vi "Read Dashboard Variables.vi"() -> ()   [LabVIEW 2019]
uses:
  <vilib>/Rock Robotics/Network Tables/NT Read Number.vi
  Framework/Robot Global Data.vi
  <vilib>/Rock Robotics/Network Tables/NT Read String.vi
  <vilib>/Rock Robotics/Network Tables/NT Read Boolean.vi
panel:
  out "Speed Rate at 2 inches":dbl
  out "Speed Rate at 6 inches":dbl
  out "Data Logger":bool
  out "Pivot Right R":dbl=0.4
  out "Pivot Right L":dbl=0.3
  out "Pivot Left R":dbl=0.4
  out "Pivot Left L":dbl=0.3
  out "Path":string
  out "MaxSpeedSlow":dbl=0.6
  out "Intake Set Point":dbl=1.0
  out "Intake Duration":dbl=0.5
  out "Shooter Set Point":dbl=1.0
  out "Shooter Duration":dbl=0.5
  out "Transfer Set Point":dbl=0.6
  out "Transfer Duration":dbl=0.5
  out "Control Panel Set Point":dbl=0.6
  out "Control Panel Duration":dbl=5.5
  out "Control Panel Color Set Point":dbl=0.3
  out "Control Panel Color Duration":dbl=4.0
  out "MaxDrive":dbl(slide)=1.0 min=0.0 max=1.0 step=0.01 scale=0.0..1.0
  out "DriveK":dbl(slide)=0.5 min=0.0 max=1.0 step=0.05 scale=0.0..1.0
  out "Limelight Goal Area":dbl(slide)=1.91 min=0.1 max=2.5 step=0.25 scale=0.0..2.5
  out "MinSteerCommand":dbl(slide)=0.2717391304347826 min=0.0 max=0.5 step=0.05 scale=0.0..0.5
  out "SteeringK":dbl(slide)=0.025362318840579712 min=0.0 max=0.25 step=0.01 scale=0.0..0.25
  out "AimDeadband":dbl=0.1 min=0.0 max=10.0 step=0.25
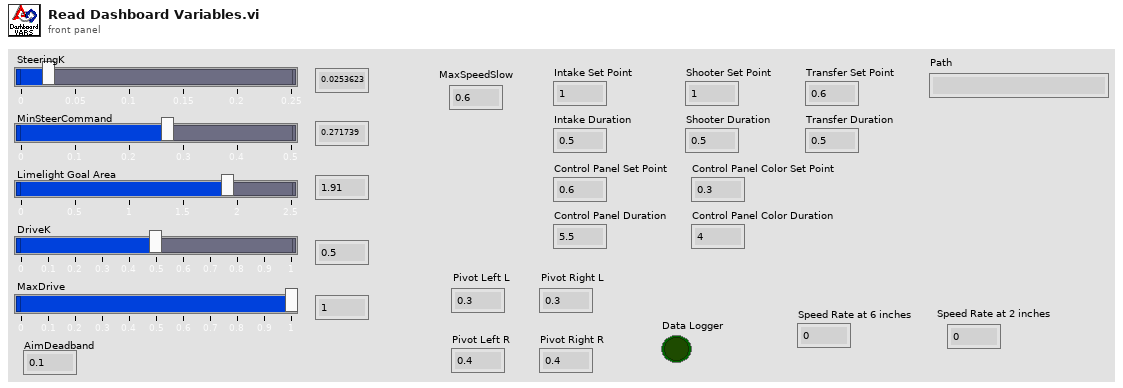
[diagram p1: front panel]
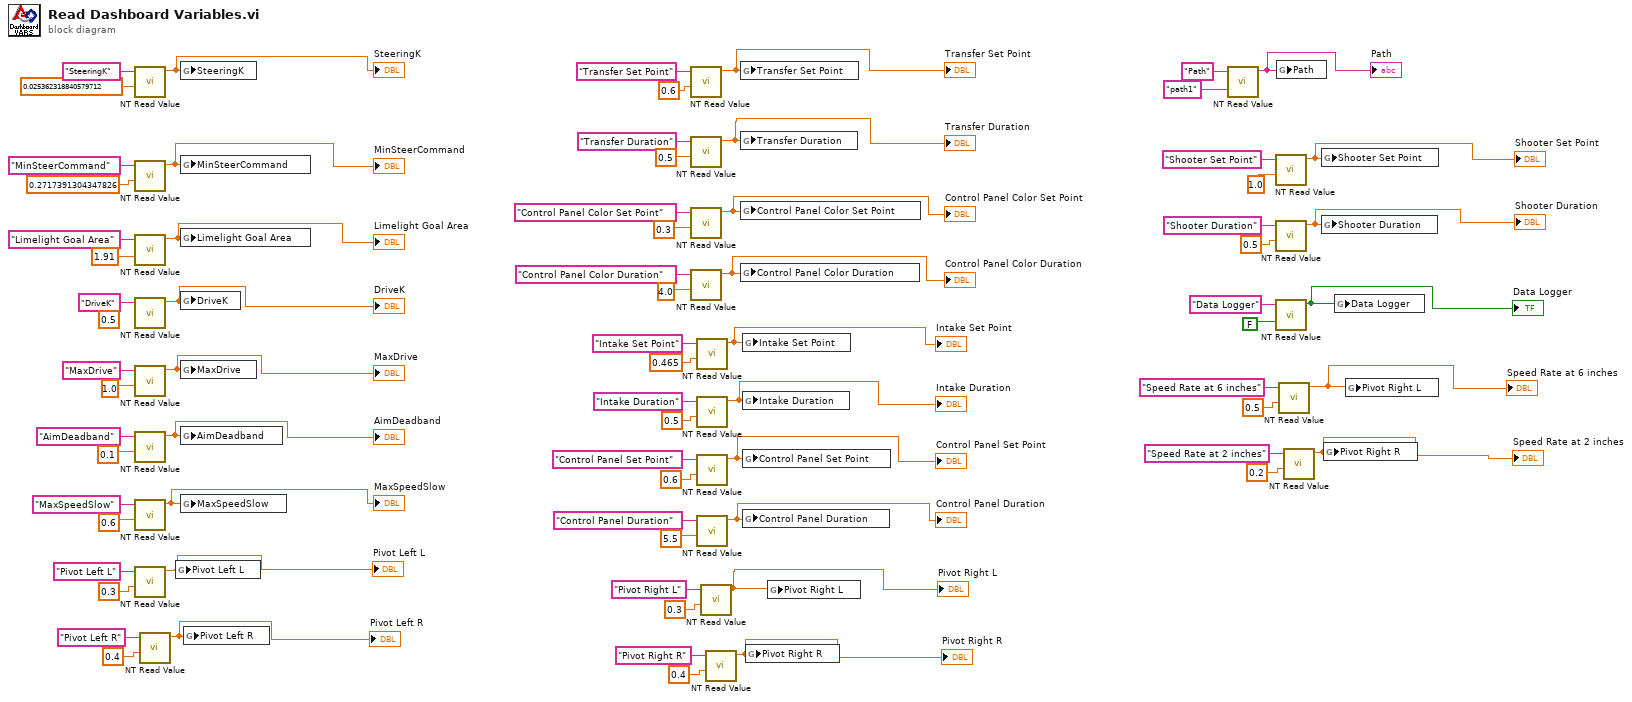
[diagram p0: block diagram]
diagram:
  (unwired) 0.5 ("DriveK")
  n1 = call-poly <vilib>:"NT Read Value.vi"("Default Value"=0.025362318840579712 ("SteeringK"), "Name"="SteeringK") -> ("Numeric"=w37:dbl)  [unwired: 8 in, 1 out]
  "SteeringK" <- w37
  n2 = call-poly <vilib>:"NT Read Value.vi"("Default Value"=0.2717391304347826 ("MinSteerCommand"), "Name"="MinSteerCommand") -> ("Numeric"=w22:dbl)  [unwired: 8 in, 1 out]
  "MinSteerCommand" <- w22
  n3 = call-poly <vilib>:"NT Read Value.vi"("Default Value"=1.91 ("Limelight Goal Area"), "Name"="Limelight Goal Area") -> ("Numeric"=w36:dbl)  [unwired: 8 in, 1 out]
  "Limelight Goal Area" <- w36
  n4 = call-poly <vilib>:"NT Read Value.vi"("Name"="DriveK") -> ("Numeric"=w35:dbl)  [unwired: 9 in, 1 out]
  "DriveK" <- w35
  n5 = call-poly <vilib>:"NT Read Value.vi"("Default Value"=1.0 ("MaxDrive"), "Name"="MaxDrive") -> ("Numeric"=w34:dbl)  [unwired: 8 in, 1 out]
  "MaxDrive" <- w34
  n6 = call-poly <vilib>:"NT Read Value.vi"("Default Value"=0.1 ("AimDeadband"), "Name"="AimDeadband") -> ("Numeric"=w33:dbl)  [unwired: 8 in, 1 out]
  "AimDeadband" <- w33
  n7 = call-poly <vilib>:"NT Read Value.vi"("Default Value"=0.6 ("MaxSpeedSlow"), "Name"="MaxSpeedSlow") -> ("Numeric"=w32:dbl)  [unwired: 8 in, 1 out]
  "MaxSpeedSlow" <- w32
  n8 = call-poly <vilib>:"NT Read Value.vi"("Default Value"=0.3 ("Pivot Left"), "Name"="Pivot Left L") -> ("Numeric"=w17:dbl)  [unwired: 8 in, 1 out]
  "Pivot Left L" <- w17
  n9 = call-poly <vilib>:"NT Read Value.vi"("Default Value"=0.4 ("Pivot right"), "Name"="Pivot Left R") -> ("Numeric"=w16:dbl)  [unwired: 8 in, 1 out]
  "Pivot Left R" <- w16
  n10 = global write "Robot Global Data.vi" "Pivot Left L"(w17) -> ()
  n11 = global write "Robot Global Data.vi" "SteeringK"(w37) -> ()
  n12 = global write "Robot Global Data.vi" "MinSteerCommand"(w22) -> ()
  n13 = global write "Robot Global Data.vi" "Limelight Goal Area"(w36) -> ()
  n14 = global write "Robot Global Data.vi" "DriveK"(w35) -> ()
  n15 = global write "Robot Global Data.vi" "MaxDrive"(w34) -> ()
  n16 = global write "Robot Global Data.vi" "AimDeadband"(w33) -> ()
  n17 = global write "Robot Global Data.vi" "MaxSpeedSlow"(w32) -> ()
  n18 = global write "Robot Global Data.vi" "Pivot Left R"(w16) -> ()
  n19 = call-poly <vilib>:"NT Read Value.vi"("Default Value"=0.6 ("Transfer Set Point"), "Name"="Transfer Set Point") -> ("Numeric"=w26:dbl)  [unwired: 8 in, 1 out]
  "Transfer Set Point" <- w26
  n20 = call-poly <vilib>:"NT Read Value.vi"("Default Value"=0.5 ("Transfer Duration"), "Name"="Transfer Duration") -> ("Numeric"=w25:dbl)  [unwired: 8 in, 1 out]
  "Transfer Duration" <- w25
  n21 = call-poly <vilib>:"NT Read Value.vi"("Default Value"=0.3 ("Control Panel Color Set Point"), "Name"="Control Panel Color Set Point") -> ("Numeric"=w24:dbl)  [unwired: 8 in, 1 out]
  "Control Panel Color Set Point" <- w24
  n22 = call-poly <vilib>:"NT Read Value.vi"("Default Value"=4.0 ("Control Panel Color Duration"), "Name"="Control Panel Color Duration") -> ("Numeric"=w23:dbl)  [unwired: 8 in, 1 out]
  "Control Panel Color Duration" <- w23
  n23 = call-poly <vilib>:"NT Read Value.vi"("Default Value"=0.465 ("Intake Set Point"), "Name"="Intake Set Point") -> ("Numeric"=w21:dbl)  [unwired: 8 in, 1 out]
  "Intake Set Point" <- w21
  n24 = call-poly <vilib>:"NT Read Value.vi"("Default Value"=0.5 ("Intake Duration"), "Name"="Intake Duration") -> ("Numeric"=w31:dbl)  [unwired: 8 in, 1 out]
  "Intake Duration" <- w31
  n25 = call-poly <vilib>:"NT Read Value.vi"("Default Value"=0.6 ("Control Panel Set Point"), "Name"="Control Panel Set Point") -> ("Numeric"=w30:dbl)  [unwired: 8 in, 1 out]
  "Control Panel Set Point" <- w30
  n26 = call-poly <vilib>:"NT Read Value.vi"("Default Value"=5.5 ("Control Panel Duration"), "Name"="Control Panel Duration") -> ("Numeric"=w29:dbl)  [unwired: 8 in, 1 out]
  "Control Panel Duration" <- w29
  n27 = call-poly <vilib>:"NT Read Value.vi"("Default Value"=0.3 ("Pivot Left"), "Name"="Pivot Right L") -> ("Numeric"=w10:dbl)  [unwired: 8 in, 1 out]
  "Pivot Right L" <- w10
  n28 = call-poly <vilib>:"NT Read Value.vi"("Default Value"=0.4 ("Pivot right"), "Name"="Pivot Right R") -> ("Numeric"=w11:dbl)  [unwired: 8 in, 1 out]
  "Pivot Right R" <- w11
  n29 = global write "Robot Global Data.vi" "Transfer Set Point"(w26) -> ()
  n30 = global write "Robot Global Data.vi" "Transfer Duration"(w25) -> ()
  n31 = global write "Robot Global Data.vi" "Control Panel Color Set Point"(w24) -> ()
  n32 = global write "Robot Global Data.vi" "Control Panel Color Duration"(w23) -> ()
  n33 = global write "Robot Global Data.vi" "Intake Set Point"(w21) -> ()
  n34 = global write "Robot Global Data.vi" "Intake Duration"(w31) -> ()
  n35 = global write "Robot Global Data.vi" "Control Panel Set Point"(w30) -> ()
  n36 = global write "Robot Global Data.vi" "Control Panel Duration"(w29) -> ()
  n37 = global write "Robot Global Data.vi" "Pivot Right R"(w11) -> ()
  n38 = global write "Robot Global Data.vi" "Pivot Right L"(w10) -> ()
  n39 = call-poly <vilib>:"NT Read Value.vi"("Default Value"="path1", "Name"="Path") -> ("String"=w18:string)  [unwired: 8 in, 1 out]
  "Path" <- w18
  n40 = call-poly <vilib>:"NT Read Value.vi"("Default Value"=1.0 ("Shooter Set Point"), "Name"="Shooter Set Point") -> ("Numeric"=w28:dbl)  [unwired: 8 in, 1 out]
  "Shooter Set Point" <- w28
  n41 = call-poly <vilib>:"NT Read Value.vi"("Default Value"=0.5 ("Shooter Duration"), "Name"="Shooter Duration") -> ("Numeric"=w27:dbl)  [unwired: 8 in, 1 out]
  "Shooter Duration" <- w27
  n42 = call-poly <vilib>:"NT Read Value.vi"("Default Value"=FALSE, "Name"="Data Logger") -> ("Boolean"=w7:bool)  [unwired: 8 in, 1 out]
  "Data Logger" <- w7
  n43 = global write "Robot Global Data.vi" "Path"(w18) -> ()
  n44 = call-poly <vilib>:"NT Read Value.vi"("Default Value"=0.5 ("Pivot Left"), "Name"="Speed Rate at 6 inches") -> ("Numeric"=w1:dbl)  [unwired: 8 in, 1 out]
  "Speed Rate at 6 inches" <- w1
  n45 = call-poly <vilib>:"NT Read Value.vi"("Default Value"=0.2 ("Pivot right"), "Name"="Speed Rate at 2 inches") -> ("Numeric"=w2:dbl)  [unwired: 8 in, 1 out]
  "Speed Rate at 2 inches" <- w2
  n46 = global write "Robot Global Data.vi" "Shooter Set Point"(w28) -> ()
  n47 = global write "Robot Global Data.vi" "Shooter Duration"(w27) -> ()
  n48 = global write "Robot Global Data.vi" "Pivot Right R"(w2) -> ()
  n49 = global write "Robot Global Data.vi" "Data Logger"(w7) -> ()
  n50 = global write "Robot Global Data.vi" "Pivot Right L"(w1) -> ()
